vi "CSVLogger.vi"() -> ()   [LabVIEW 2026]
panel:
  in  "Status":string
  in  "Voltage":dbl
  in  "Humidity":dbl
  in  "Temperature":dbl
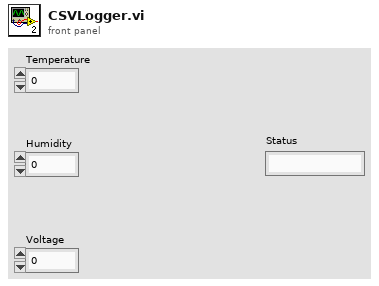
[diagram p1: front panel]
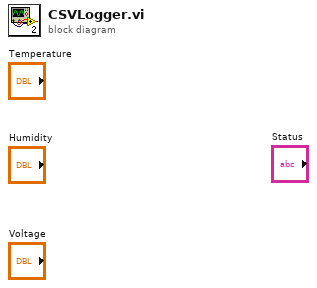
[diagram p0: block diagram]
diagram:
